vi "Rising Edge True.vi"(11 "Input":bool) -> (3 "Output":bool)   [LabVIEW 2015]
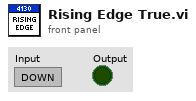
[diagram p1: front panel]
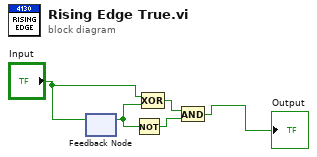
[diagram p0: block diagram]
diagram:
  n1 = feedback #1() -> (w2:bool)  [unwired: 1 in]
  n2 = feedback-in #1("Input") -> ()
  n3 = Not(x=w2) -> (.not. x?=w4:bool)
  n4 = Compound Arithmetic op=XOR("Input", w2) -> (w3:bool)
  n5 = And(x=w3, y=w4) -> (x .and. y?=→"Output":bool)
